vi "from_item.vi"(8 "error in (no error)":errorcluster, 10 "item_ref":u64) -> (0 "error out":errorcluster, 3 "Value out":refnum<class "Value.lvclass">)   [LabVIEW 2020, in "toml_edit.lvlib" / "Value.lvclass"]
uses:
  Value.lvclass
  Value.lvclass/Value.ctl
  dragon_toml_64.dll
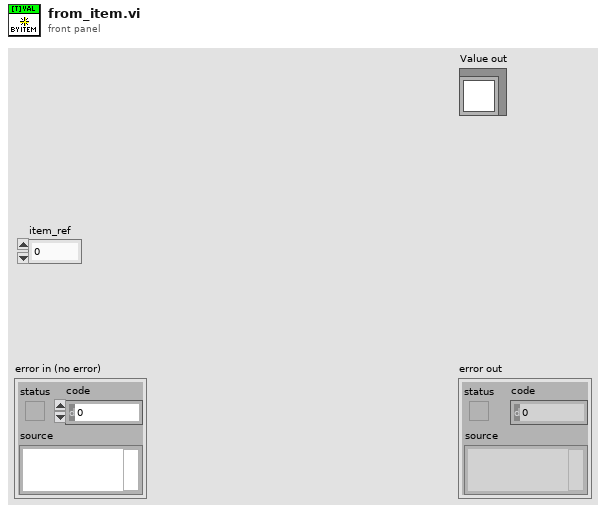
[diagram p1: front panel]
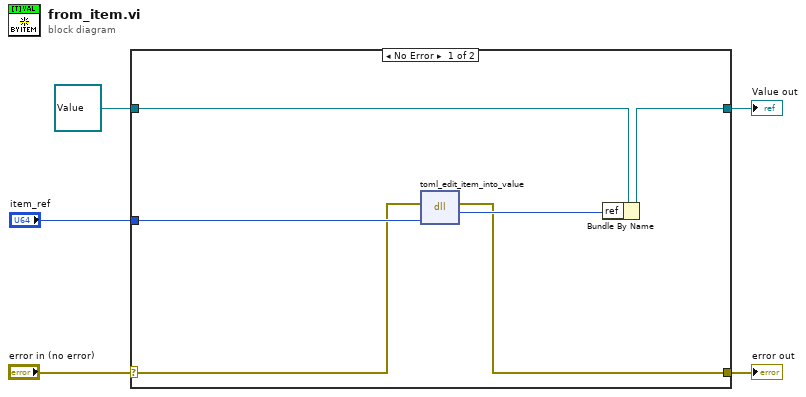
[diagram p0: block diagram]
diagram:
  n1 = case shown="No Error" "error in (no error)" {
    selector: "error in (no error)" -> [w7 w13]
    tunnel: [w6 w13] -> w4
    tunnel: [w9 w12] -> w2
    tunnel: refnum<class "Value.lvclass"> refnum ("Value in") -> [w11 w12]
    tunnel: "item_ref" -> [w10 _]
    frame No Error {
      n2 = dll-call lib="C:/Projects/labview-project-load-tools/rust_src/toml_edit_dll/lv_src/dragon_toml_*.dll" fn="toml_edit_item_into_value"(error in=w7, "item"=w10) -> (error out=w6:errorcluster, "value"=w8:u64)  [unwired: 3 in, 1 out]
      n3 = Bundle By Name(cluster=w11, "ref"=w8) -> (w9:refnum<class "Value.lvclass">)
    }
    frame Error {
    }
  }
  "error out" <- w4
  "Value out" <- w2
